vi "waitTrig.vi"(3 "Trigger\nextern":bool) -> (0 "ESCKey":bool, 1 "SpaceKey":bool)   [LabVIEW 2015]
uses:
  ESLSCDLL.dll
panel:
  in  "Numerisch 2":u8
  in  "Numerisch":u8
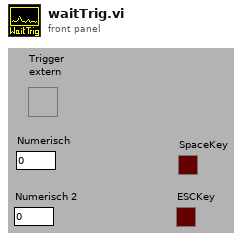
[diagram p1: front panel]
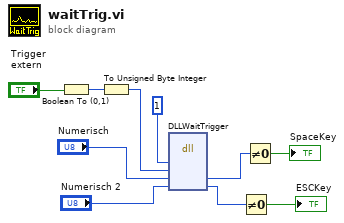
[diagram p0: block diagram]
diagram:
  n1 = Boolean To (0,1)(Boolean="Trigger\nextern") -> (0, 1=w2:i16)
  n2 = To Unsigned Byte Integer(number=w2) -> (unsigned 8bit integer=w1:u8)
  n3 = dll-call lib="C:/ENTW/PCIE/64bit/lv64/1cam/board.vis/ESLSCDLL.dll" fn="DLLWaitTrigger"("drv"=u32 1, "ExtTrig"=w1, "SpaceKey"="Numerisch", "EscapeKey"="Numerisch 2") -> ("SpaceKey"=w3:u8, "EscapeKey"=w4:u8)  [unwired: 6 in, 2 out]
  n4 = Not Equal To 0?(x=w4) -> (x != 0?=→"ESCKey":bool)
  n5 = Not Equal To 0?(x=w3) -> (x != 0?=→"SpaceKey":bool)
